vi "interpret line.vi"(8 "line":string) -> (0 "datentyp":T1, 1 "LOG":string, 2 "calibration data out":dbl[](array[numeric]), 3 "source data out":dbl[](array[numeric]))   [LabVIEW 2017, in "LicorLI7000.lvlib"]
uses:
  LicorLI7000.lvlib
  datentyp.ctl
  <vilib>/regexp/Match Regular Expression.xnode
panel:
  in  "Offset (0)":i32
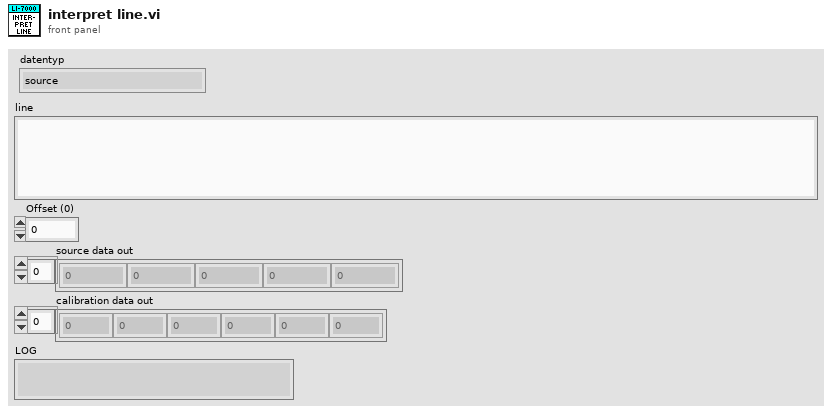
[diagram p1: front panel]
types:
  T1 = typedef "LicorLI7000.lvlib/datentyp.ctl" = enum16{"source", "calibration", "LOG"}
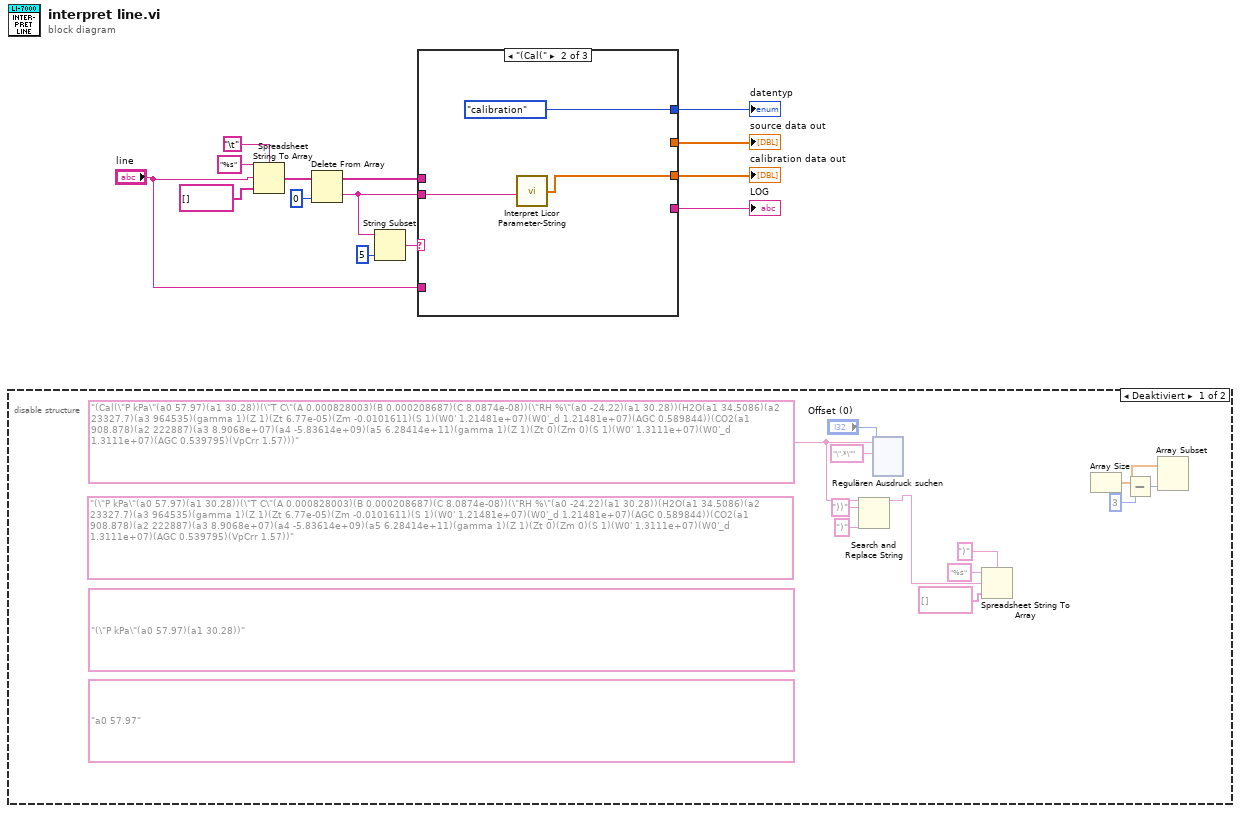
[diagram p0: block diagram]
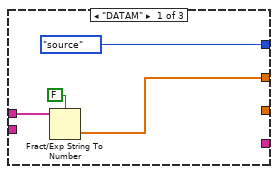
[diagram p2: hidden frame]
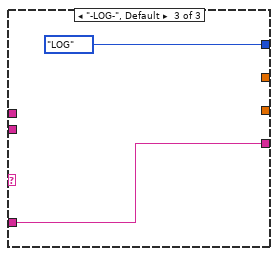
[diagram p3: hidden frame]
diagram:
  n1 = disable-structure shown="Deaktiviert" {
    frame Disabled {
      (unwired) "a0 57.97"
      (unwired) "(\"P kPa\"(a0 57.97)(a1 30.28))"
      (unwired) "(\"P kPa\"(a0 57.97)(a1 30.28))(\"T C\"(A 0.000828003)(B 0.000208687)(C 8.0874e-08))(\"RH %\"(a0 -24.22)(a1 30.28))(H2O(a1 34.5086)(a2 23327.7)(a3 964535)(gamma 1)(Z 1)(Zt 6.77e-05)(Zm -0.0101611)(S 1)(W0' 1.21481e+07)(W0'_d 1.21481e+07)(AGC 0.589844))(CO2(a1 908.878)(a2 222887)(a3 8.9068e+07)(a4 -5.83614e+09)(a5 6.28414e+11)(gamma 1)(Z 1)(Zt 0)(Zm 0)(S 1)(W0' 1.3111e+07)(W0'_d 1.3111e+07)(AGC 0.539795)(VpCrr 1.57))"
      w26 = "(Cal(\"P kPa\"(a0 57.97)(a1 30.28))(\"T C\"(A 0.000828003)(B 0.000208687)(C 8.0874e-08))(\"RH %\"(a0 -24.22)(a1 30.28))(H2O(a1 34.5086)(a2 23327.7)(a3 964535)(gamma 1)(Z 1)(Zt 6.77e-05)(Zm -0.0101611)(S 1)(W0' 1.21481e+07)(W0'_d 1.21481e+07)(AGC 0.589844))(CO2(a1 908.878)(a2 222887)(a3 8.9068e+07)(a4 -5.83614e+09)(a5 6.28414e+11)(gamma 1)(Z 1)(Zt 0)(Zm 0)(S 1)(W0' 1.3111e+07)(W0'_d 1.3111e+07)(AGC 0.539795)(VpCrr 1.57)))"
      n2 = Search and Replace String(input string=w26, search string="))" ("Such-String"), replace string=")" ("Ersetzungs-String (\"\")")) -> (result string=w20:string)  [unwired: 5 in, 3 out]
      n3 = xnode "Regulären Ausdruck suchen"("input string"=w26, "regular expression"="\".*\"" ("Regulärer Ausdruck"), "offset (0)"="Offset (0)") -> ()  [unwired: 3 in, 5 out]
      n4 = Spreadsheet String To Array(delimiter (Tab)=")" ("Trennzeichen (Tabulator)"), format string="%s" ("Format-String"), spreadsheet string=w20, array type (2D Dbl)=string[] []) -> (array=w19:string[])
      n5 = Array Size(array=w18) -> (size(s)=w17:i32)
      n6 = Subtract(x=w17, y=3) -> (x-y=w15:i32)
      n7 = Array Subset(length=w15) -> (array=w18:dbl[])  [unwired: 1 in, 1 out]
    }
    frame Enabled {
    }
  }
  n8 = Spreadsheet String To Array(delimiter (Tab)="\t", format string="%s", spreadsheet string="line", array type (2D Dbl)=string[] []) -> (array=w4:string[])
  n9 = Delete From Array(array=w4, index=0 ("Index")) -> (deleted portion=w1:string, array with subset deleted=w3:string[])  [unwired: 1 in]
  n10 = String Subset(string=w1, length (rest)=5 ("Länge (Rest)")) -> (substring=w13:string)  [unwired: 1 in]
  n11 = case shown="\"(Cal(\"" w13 {
    tunnel: [_ w145 _] -> w8
    tunnel: [w141 _ _] -> w9
    tunnel: w3 -> [w140 _ _]
    tunnel: [_ _ w147] -> w5
    tunnel: [datentyp."source" datentyp."calibration" datentyp."LOG"] -> w7
    tunnel: "line" -> [_ _ w147]
    tunnel: w1 -> [_ w144 _]
    frame "DATAM" {
      n12 = Fract/Exp String To Number(use system decimal point (T)=FALSE ("Systemdezimalzeichen verwenden (T)"), string=w140) -> (number=w141:dbl[])  [unwired: 2 in, 1 out]
    }
    frame "(Cal(" {
      n13 = call "Interpret Licor Parameter-String.vi"("Tabellen-String"=w144) -> ("Parameter"=w145:dbl[])  [unwired: 14 in]
    }
    frame "-LOG-", Default {
    }
  }
  "calibration data out" <- w8
  "source data out" <- w9
  "datentyp" <- w7
  "LOG" <- w5
